vi "ErrorConsole.vi"(8 "error in (no error)":errorcluster) -> (0 "error out":errorcluster)   [LabVIEW 2013, in "ErrorConsoleLib.lvlib"]
doc: "Error handler handles all categories of error of ATM Application."
uses:
  ErrorConsoleLib.lvlib
  PrivateControls/ErrorConsole_QueueDriver.ctl
  MainVI/TopLevelController/Private Controls/Terminate.ctl
  MainVI/TopLevelController/ToplevelControllerLibrary.lvlib
panel:
  # "Error handler handles all categories of error of ATM Application."
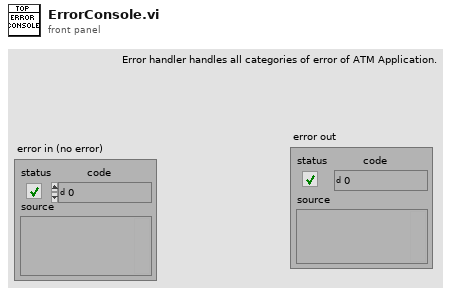
[diagram p1: front panel]
types:
  T1 = enum16{"Create Event", "Generate Event", "Destroy Event"}
  T2 = typedef "ErrorConsoleLib.lvlib/ErrorConsole_QueueDriver.ctl" = enum16{"Default", "Init", "Enqueue", "Dequeue", "ReleaseQueue", "Exit"}
  T3 = typedef "ToplevelControllerLibrary.lvlib/Terminate.ctl" = enum16{"Update UserConsole", "Update DisplayConsole", "ReInit"}
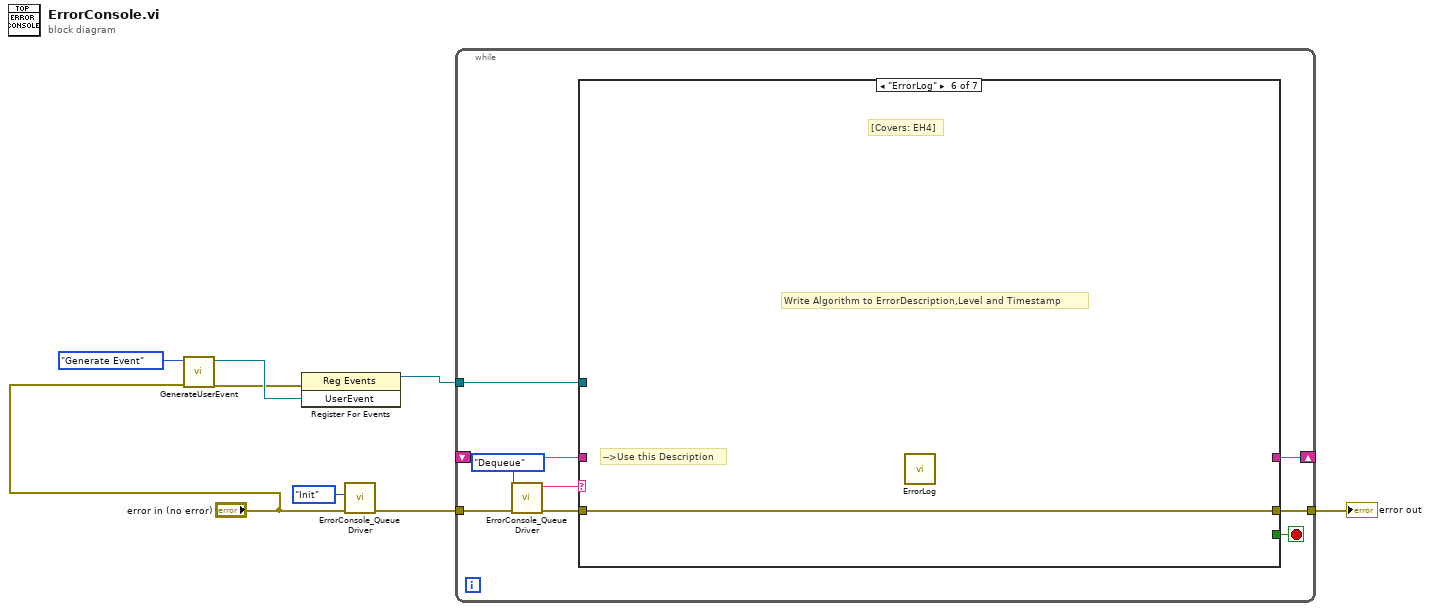
[diagram p0: block diagram]
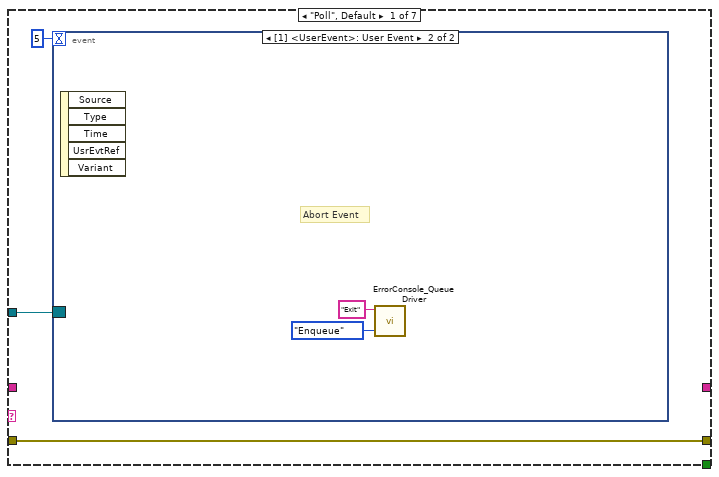
[diagram p2: hidden frame]
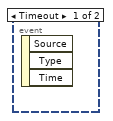
[diagram p3: hidden frame]
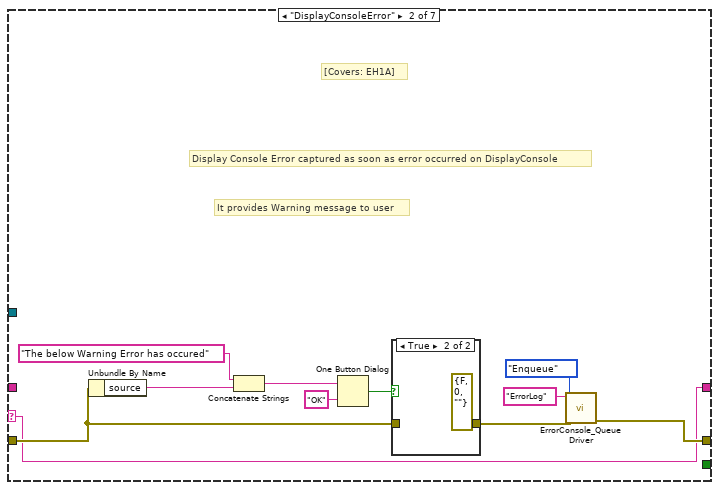
[diagram p4: hidden frame]
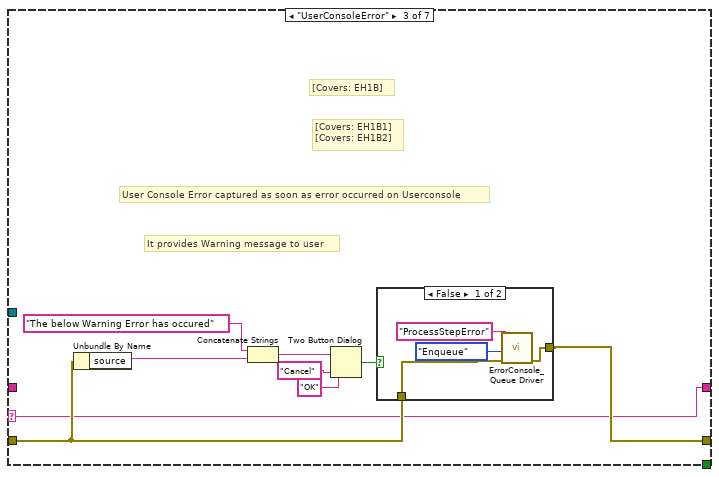
[diagram p6: hidden frame]
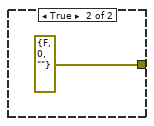
[diagram p7: hidden frame]
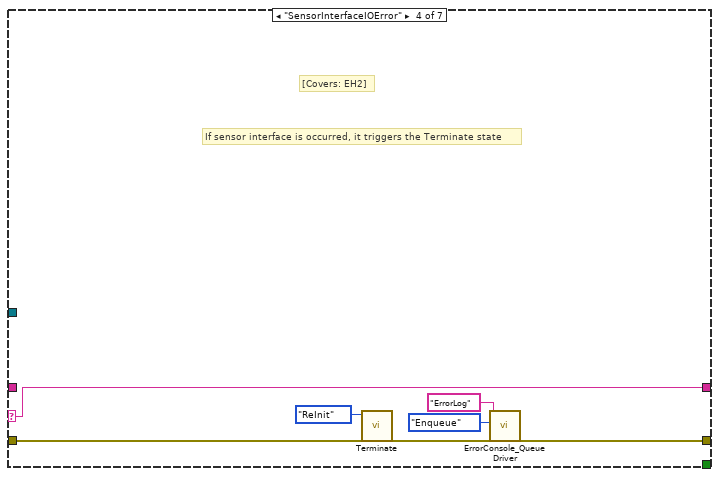
[diagram p8: hidden frame]
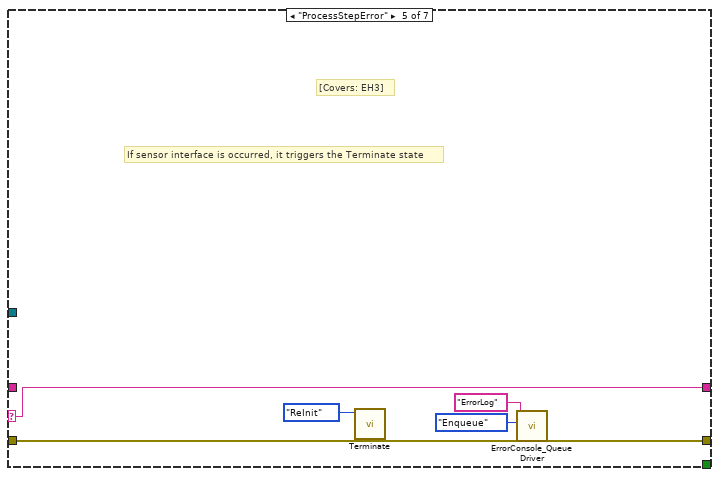
[diagram p9: hidden frame]
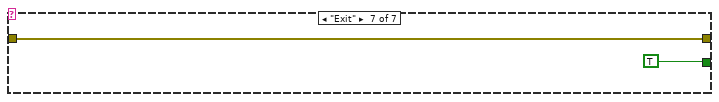
[diagram p10: hidden frame]
diagram:
  n1 = call "GenerateUserEvent.vi"("error in (no error)"="error in (no error)", "Event Actions"=T1."Generate Event") -> ("error out"=w3:errorcluster, "UserEvent"=w4:refnum<user-event>)  [unwired: 8 in]
  n2 = register-events(error in=w3, w4) -> (reference out=w2:refnum<event-registration>)  [unwired: 1 in, 1 out]
  n3 = call "ErrorConsole_Queue Driver.vi"("error in (no error)"="error in (no error)", "State"=ErrorConsole_QueueDriver."Init") -> ("error out"=w7:errorcluster)  [unwired: 8 in, 1 out]
  n4 = while {
    tunnel: w7 -> [w16]
    tunnel: [w17] -> w8
    shift-right: [w12] -> _
    shift-left: _ -> [w11]
    tunnel: w2 -> [w10]
    stop <- w9 stop-if-true
    n5 = call "ErrorConsole_Queue Driver.vi"("error in (no error)"=w16, "State"=ErrorConsole_QueueDriver."Dequeue") -> ("error out"=w15:errorcluster, "DeQ"=w14:string)  [unwired: 8 in]
    n6 = case shown="\"ErrorLog\"" w14 {
      selector: w14 -> [_ w23 w36 w50 w55 _ _]
      tunnel: w15 -> [w20 w24 w37 w54 w59 w60 w62]
      tunnel: [w20 w26 w38 w54 w59 w60 w62] -> w17
      tunnel: [_ w23 w36 w50 w55 _ _] -> w12
      tunnel: w11 -> [_ _ _ _ _ _ _]
      tunnel: w10 -> [w18 _ _ _ _ _ _]
      tunnel: [_ _ _ _ _ _ TRUE] -> w9
      frame "Poll", Default {
        n7 = event shown="[1] <UserEvent>: User Event" {
          selector: w18 -> [_ _]
          dyn-events: _ -> [_ _]
          timeout: 5 -> [_ _]
          event Timeout {
            n8 = event-data() -> ()  [unwired: 1 in, 3 out]
          }
          event User Event {
            # "Abort Event"
            n9 = event-data() -> ()  [unwired: 1 in, 5 out]
            n10 = call "ErrorConsole_Queue Driver.vi"("State"=ErrorConsole_QueueDriver."Enqueue", "EnQ"="Exit") -> ()  [unwired: 8 in, 2 out]
          }
        }
      }
      frame "DisplayConsoleError" {
        # "It provides Warning message to user"
        # "Display Console Error captured as soon as error occurred on DisplayConsole"
        # "[Covers: EH1A]"
        n11 = Unbundle By Name(w24) -> ("source"=w32:string)
        n12 = Concatenate Strings("The below Warning Error has occured", w32) -> (w31:string)
        n13 = One Button Dialog(message=w31, button name ("OK")="OK") -> (true=w29:bool)
        n14 = case shown="True" w29 {
          tunnel: [w34 errorcluster {"status"=FALSE, "code"=0, "source"=""} ("error constant")] -> w27
          tunnel: w24 -> [w34 _]
          frame False {
          }
          frame True {
          }
        }
        n15 = call "ErrorConsole_Queue Driver.vi"("error in (no error)"=w27, "State"=ErrorConsole_QueueDriver."Enqueue", "EnQ"="ErrorLog") -> ("error out"=w26:errorcluster)  [unwired: 7 in, 1 out]
      }
      frame "UserConsoleError" {
        # "It provides Warning message to user"
        # "User Console Error captured as soon as error occurred on Userconsole"
        # "[Covers: EH1B1] \n[Covers: EH1B2]"
        # "[Covers: EH1B]"
        n16 = Unbundle By Name(w37) -> ("source"=w43:string)
        n17 = Concatenate Strings("The below Warning Error has occured", w43) -> (w42:string)
        n18 = Two Button Dialog(message=w42, 1:"Cancel" ("button name (\"OK\")"), 2:"OK" ("T button name (\"OK\")")) -> (T button?=w40:bool)
        n19 = case shown="False" w40 {
          tunnel: [w46 errorcluster {"status"=FALSE, "code"=0, "source"=""} ("error constant")] -> w38
          tunnel: w37 -> [w45 _]
          frame False {
            n20 = call "ErrorConsole_Queue Driver.vi"("error in (no error)"=w45, "State"=ErrorConsole_QueueDriver."Enqueue", "EnQ"="ProcessStepError") -> ("error out"=w46:errorcluster)  [unwired: 7 in, 1 out]
          }
          frame True {
          }
        }
      }
      frame "SensorInterfaceIOError" {
        # "If sensor interface is occurred, it triggers the Terminate state"
        # "[Covers: EH2]"
        n21 = call "Terminate.vi"("Terminate"=Terminate."ReInit") -> ()  [unwired: 11 in]
        n22 = call "ErrorConsole_Queue Driver.vi"("State"=ErrorConsole_QueueDriver."Enqueue", "EnQ"="ErrorLog") -> ()  [unwired: 8 in, 2 out]
      }
      frame "ProcessStepError" {
        # "If sensor interface is occurred, it triggers the Terminate state"
        # "[Covers: EH3]"
        n23 = call "Terminate.vi"("Terminate"=Terminate."ReInit") -> ()  [unwired: 11 in]
        n24 = call "ErrorConsole_Queue Driver.vi"("State"=ErrorConsole_QueueDriver."Enqueue", "EnQ"="ErrorLog") -> ()  [unwired: 8 in, 2 out]
      }
      frame "ErrorLog" {
        # "-->Use this Description"
        # "Write Algorithm to ErrorDescription,Level and Timestamp"
        # "[Covers: EH4]"
        n25 = call "ErrorLog.vi"() -> ()  [unwired: 12 in]
      }
      frame "Exit" {
      }
    }
  }
  "error out" <- w8
